vi "LogToInflux.vi"(3 "error in (no error)":errorcluster, 4 "InfluxDB Info":T1, 5 "InfluxDB Line Protocol":string, 6 "InfluxDB Address":string) -> (0 "error out":errorcluster, 1 "InfluxDB":bool, 2 "Rejected Items":string)   [LabVIEW 2013, in "ovenCtrl.lvlib"]
uses:
  ovenCtrl.lvlib
panel:
  # "Outputs"
  # "Inputs"
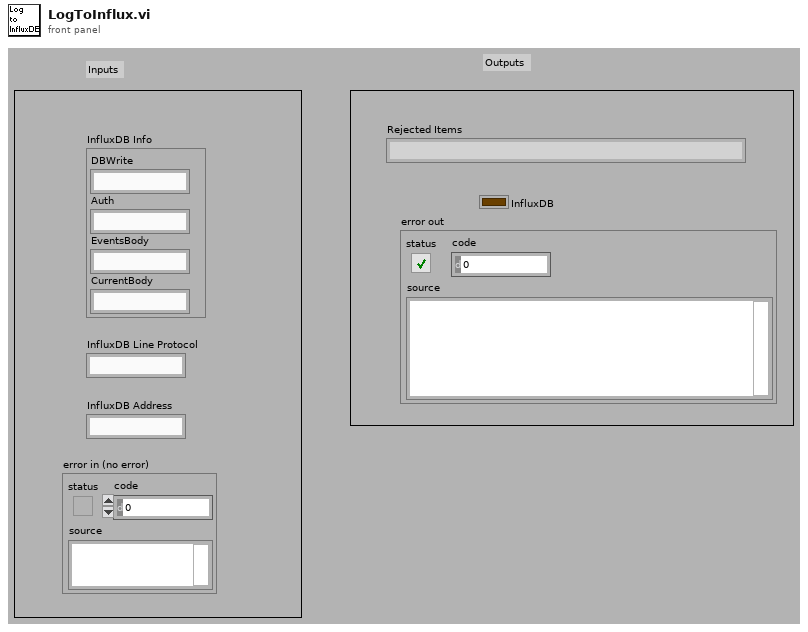
[diagram p1: front panel]
types:
  T1 = cluster{"DBWrite":string, "Auth":string, "EventsBody":string, "CurrentBody":string}
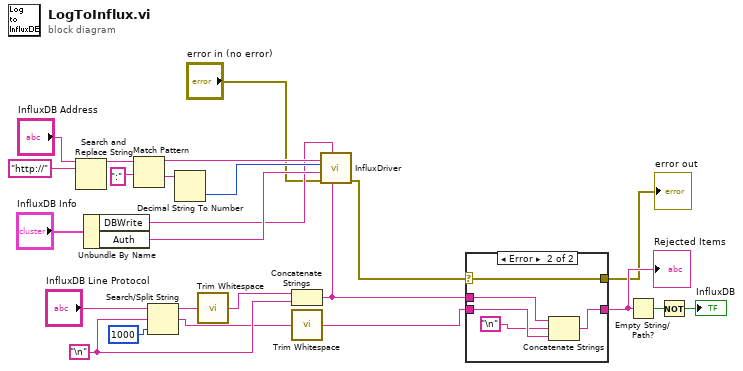
[diagram p0: block diagram]
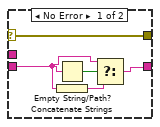
[diagram p2: hidden frame]
diagram:
  w12 = "\n"
  n1 = Search and Replace String(input string="InfluxDB Address", search string="http://" ("substring (\"\")")) -> (result string=w24:string)  [unwired: 6 in, 3 out]
  n2 = Unbundle By Name("InfluxDB Info") -> ("DBWrite"=w13:string, "Auth"=w14:string)
  n3 = Match Pattern(string=w24, regular expression=":") -> (before substring=w16:string, after substring=w21:string)  [unwired: 1 in, 2 out]
  n4 = Search/Split String(string="InfluxDB Line Protocol", search string/char (-)=w12, offset (0)=1000) -> (substring before match=w10:string, match + rest of string=w7:string)  [unwired: 1 out]
  n5 = Decimal String To Number(string=w21) -> (number=w15:i32)  [unwired: 2 in, 1 out]
  n6 = call <vilib>:"Trim Whitespace.vi"("string"=w10) -> ("trimmed string"=w9:string)  [unwired: 1 in]
  n7 = Concatenate Strings(w9, w12) -> (w6:string)
  n8 = call <vilib>:"Trim Whitespace.vi"("string"=w7) -> ("trimmed string"=w5:string)  [unwired: 1 in]
  n9 = call "InfluxDriver.vi"("body"=w6, "dbwrite"=w13, "error in (no error)"="error in (no error)", "authorization"=w14, "remote port"=w15, "InfluxDB Address"=w16) -> ("error out"=w4:errorcluster)  [unwired: 4 in, 1 out]
  n10 = case shown="Error" w4 {
    selector: w4 -> [w29 w30]
    tunnel: w6 -> [_ w34]
    tunnel: [w27 w33] -> w3
    tunnel: w5 -> [w26 w32]
    tunnel: [w29 w30] -> w1
    frame No Error {
      n11 = Empty String/Path?(string/path=w26) -> (empty?=w28:bool)
      n12 = Concatenate Strings(w26) -> (w25:string)
      n13 = Select(t=w26, s=w28, f=w25) -> (s? t:f=w27:string)
    }
    frame Error {
      n14 = Concatenate Strings(w34, "\n", w32) -> (w33:string)
    }
  }
  "Rejected Items" <- w3
  "error out" <- w1
  n15 = Empty String/Path?(string/path=w3) -> (empty?=w18:bool)
  n16 = Not(x=w18) -> (.not. x?=→"InfluxDB":bool)
